vi "Update Data Plot.vi"(6 "Sample Rate (sec/sample)":dbl, 8 "Time interval (s)":i32, 9 "Instrument State":T2, 10 "History length":i32=172800, 11 "Graph History Arrays in":T1) -> (0 "Updated Plot History":cluster{timestamp[], dbl[]}[](array[cluster]), 3 "Graph History Arrays out":T1)   [LabVIEW 2020, in "Polar Bear Plus All-in-One Plugin.lvlib"]
uses:
  Polar Bear Plus All-in-One Plugin.lvlib
  Instrument Manager/Instrument State.ctl
  <instrlib>/RxnRover/Driver Polar Bear Plus/heater_parent/heater_parent.lvclass
  Data Display Loop Data.ctl
  Instrument Manager/Instrument Manager.lvlib
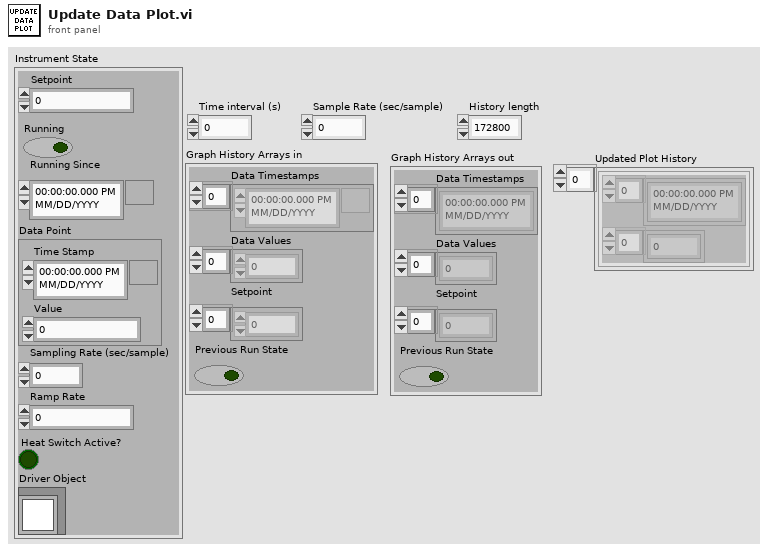
[diagram p1: front panel]
types:
  T1 = typedef "Polar Bear Plus All-in-One Plugin.lvlib/Data Display Loop Data.ctl" = cluster{"Data Timestamps":timestamp[], "Data Values":dbl[], "Setpoint":dbl[], "Previous Run State":bool}
  T2 = typedef "Polar Bear Plus All-in-One Plugin.lvlib/Instrument Manager.lvlib/Instrument State.ctl" = cluster{"Setpoint":dbl, "Running":bool, "Running Since":timestamp, "Data Point":cluster{"Time Stamp":timestamp, "Value":dbl}, "Sampling Rate (sec/sample)":dbl, "Ramp Rate":dbl, "Heat Switch Active?":bool, "Driver Object":refnum<class "heater_parent.lvclass">}
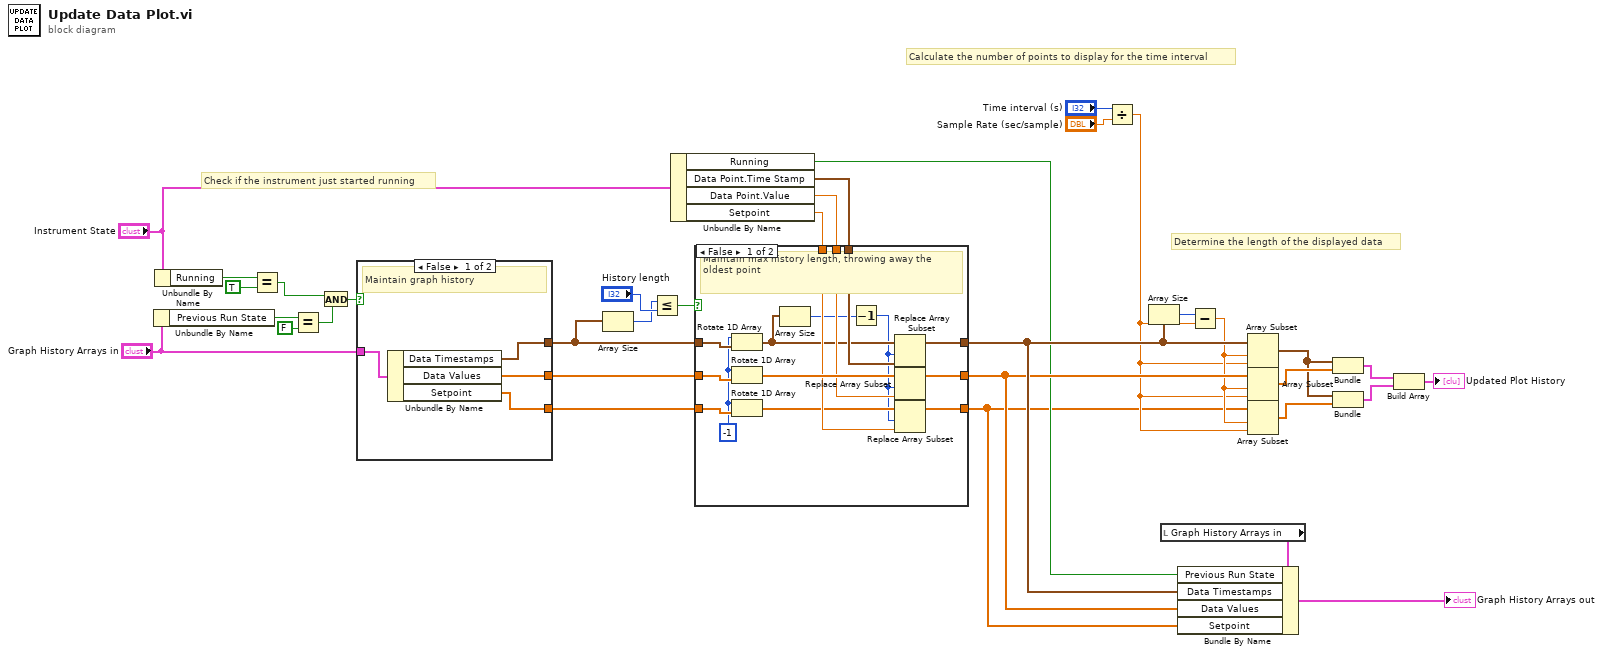
[diagram p0: block diagram]
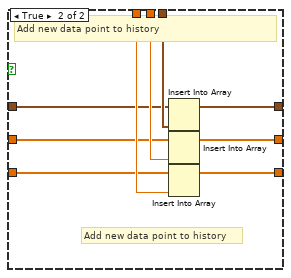
[diagram p2: hidden frame]
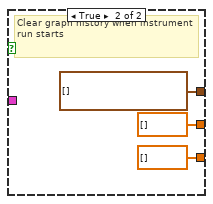
[diagram p3: hidden frame]
diagram:
  # "Check if the instrument just started running"
  # "Calculate the number of points to display for the time interval"
  # "Determine the length of the displayed data"
  n1 = Unbundle By Name("Graph History Arrays in") -> ("Previous Run State"=w19:bool)
  n2 = Unbundle By Name("Instrument State") -> ("Running"=w27:bool)
  n3 = Equal?(x=w27, y=TRUE) -> (x = y?=w15:bool)
  n4 = Equal?(x=w19, y=FALSE) -> (x = y?=w16:bool)
  n5 = And(x=w15, y=w16) -> (x .and. y?=w17:bool)
  n6 = case shown="False" w17 {
    tunnel: "Graph History Arrays in" -> [w39 _]
    tunnel: [w38 dbl[] [] ("Data Values")] -> w21
    tunnel: [w37 timestamp[] [] ("Data Timestamps")] -> w4
    tunnel: [w36 dbl[] [] ("Setpoint")] -> w14
    frame False {
      # "Maintain graph history"
      n7 = Unbundle By Name(w39) -> ("Data Timestamps"=w37:timestamp[], "Data Values"=w38:dbl[], "Setpoint"=w36:dbl[])
    }
    frame True {
      # "Clear graph history when instrument run starts"
    }
  }
  n8 = Array Size(array=w4) -> (size(s)=w2:i32)
  n9 = Less Or Equal?(x=w2, y="History length") -> (x <= y?=w1:bool)
  n10 = Unbundle By Name("Instrument State") -> ("Running"=w6:bool, "Data Point.Time Stamp"=w23:timestamp, "Data Point.Value"=w22:dbl, "Setpoint"=w28:dbl)
  n11 = case shown="False" w1 {
    tunnel: w28 -> [w52 w66]
    tunnel: [w45 w65] -> w26
    tunnel: [w44 w64] -> w25
    tunnel: w23 -> [w49 w63]
    tunnel: w22 -> [w50 w62]
    tunnel: w21 -> [w56 w61]
    tunnel: w14 -> [w55 w60]
    tunnel: [w43 w59] -> w5
    tunnel: w4 -> [w57 w58]
    frame False {
      w54 = -1
      # "Maintain max history length, throwing away the oldest point"
      n12 = Rotate 1D Array(1:w57, 2:w54) -> (0:w48:timestamp[])
      n13 = Rotate 1D Array(1:w56, 2:w54) -> (0:w53:dbl[])
      n14 = Rotate 1D Array(1:w55, 2:w54) -> (0:w51:dbl[])
      n15 = Array Size(array=w48) -> (size(s)=w47:i32)
      n16 = Decrement(x=w47) -> (x-1=w46:i32)
      n17 = Replace Array Subset(array=w48, new element=w49, index=w46) -> (w45:timestamp[])
      n18 = Replace Array Subset(array=w53, new element=w50, index=w46) -> (w44:dbl[])
      n19 = Replace Array Subset(array=w51, new element=w52, index=w46) -> (w43:dbl[])
    }
    frame True {
      # "Add new data point to history"
      # "Add new data point to history"
      n20 = Insert Into Array(array=w58, new element=w63) -> (w65:timestamp[])  [unwired: 1 in]
      n21 = Insert Into Array(array=w61, new element=w62) -> (w64:dbl[])  [unwired: 1 in]
      n22 = Insert Into Array(array=w60, new element=w66) -> (w59:dbl[])  [unwired: 1 in]
    }
  }
  n23 = Divide(x="Time interval (s)", y="Sample Rate (sec/sample)") -> (x/y=w12:dbl)
  n24 = Array Size(array=w26) -> (size(s)=w33:i32)
  n25 = local read "Graph History Arrays in"() -> (w24:T1)
  n26 = Bundle By Name(cluster=w24, "Previous Run State"=w6, "Data Timestamps"=w26, "Data Values"=w25, "Setpoint"=w5) -> (→"Graph History Arrays out":T1)
  n27 = Subtract(x=w33, y=w12) -> (x-y=w13:dbl)
  n28 = Array Subset(array=w26, index=w13, length=w12) -> (w10:timestamp[])
  n29 = Array Subset(array=w25, index=w13, length=w12) -> (w32:dbl[])
  n30 = Array Subset(array=w5, index=w13, length=w12) -> (w11:dbl[])
  n31 = Bundle(w10, w32) -> (w9:cluster{timestamp[], dbl[]})  [unwired: 1 in]
  n32 = Bundle(w10, w11) -> (w8:cluster{timestamp[], dbl[]})  [unwired: 1 in]
  n33 = Build Array(w9, w8) -> (→"Updated Plot History":cluster{timestamp[], dbl[]}[])
